vi "IsFIFOFinished_HH.vi"(1 "Measurement":T1 {"Stop Count" format="%.2f"; "Binning [s]" format="%.2f"}, 2 "Time":u32, 3 "Counts":u32, 4 "operation":enum16{"initialize", "test limit"}(ring)) -> (0 "Boolean":bool)   [LabVIEW 2009]
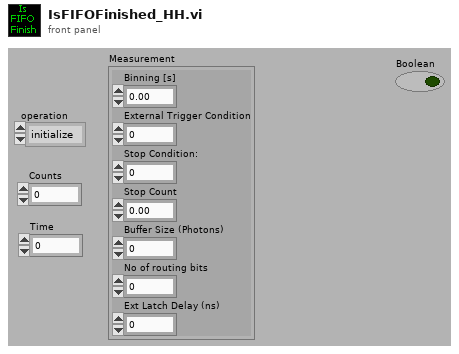
[diagram p1: front panel]
types:
  T1 = cluster{"Binning [s]":sgl, "External Trigger Condition":u16, "Stop Condition:":u16, "Stop Count":dbl, "Buffer Size (Photons)":u16, "No of routing bits":u16, "Ext Latch Delay (ns)":i16}
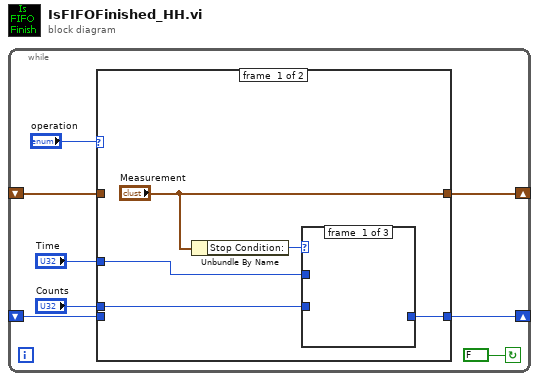
[diagram p0: block diagram]
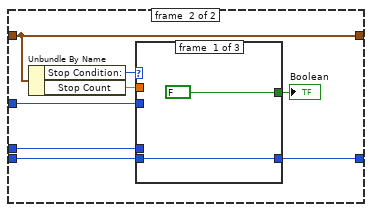
[diagram p4: hidden frame]
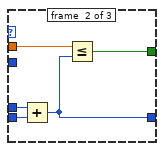
[diagram p5: hidden frame]
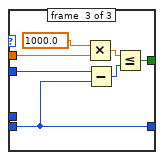
[diagram p6: hidden frame]
diagram:
  n1 = while {
    shift-right: [w6] -> _
    shift-left: _ -> [w5]
    shift-right: [w3] -> _
    shift-left: _ -> [w4]
    stop <- FALSE continue-if-true
    n2 = case shown="\"test limit\"" "operation" {
      tunnel: ["Measurement" w17] -> w6
      tunnel: w5 -> [_ w17]
      tunnel: w4 -> [_ w21]
      tunnel: [w12 w20] -> w3
      tunnel: "Counts" -> [w11 w18]
      tunnel: "Time" -> [w10 w16]
      frame #0 {
        n3 = Unbundle By Name("Measurement") -> ("Stop Condition:"=w13:u16)
        n4 = case shown="2" w13 {
          tunnel: [_ w14 w15] -> w12
          tunnel: w11 -> [_ w14 _]
          tunnel: w10 -> [_ _ w15]
          frame #0 {
          }
          frame #1 {
          }
          frame #2 {
          }
        }
      }
      frame #1 {
        n5 = Unbundle By Name(w17) -> ("Stop Condition:"=w22:u16, "Stop Count"=w19:dbl)
        n6 = case shown="1" w22 {
          tunnel: w18 -> [_ w30 _]
          tunnel: [FALSE w28 w35] -> w23
          tunnel: w21 -> [w24 w29 w37]
          tunnel: [w24 w26 w37] -> w20
          tunnel: w19 -> [_ w27 w32]
          tunnel: w16 -> [_ _ w31]
          frame #0 {
          }
          frame #1 {
            n7 = Add(x=w30, y=w29) -> (x+y=w26:u32)
            n8 = Less Or Equal?(x=w27, y=w26) -> (x <= y?=w28:bool)
          }
          frame #2 {
            n9 = Multiply(x=1000.0, y=w32) -> (x*y=w34:dbl)
            n10 = Subtract(x=w31, y=w37) -> (x-y=w36:u32)
            n11 = Less Or Equal?(x=w34, y=w36) -> (x <= y?=w35:bool)
          }
        }
        "Boolean" <- w23
      }
    }
  }
